vi "Write Registration Complete.vi"(8 "error in":errorcluster, 10 "Registration Complete":bool, 11 "File Actor in":refnum<class "File Actor.lvclass">) -> (0 "error out":errorcluster, 3 "File Actor out":refnum<class "File Actor.lvclass">)   [LabVIEW 2017, in "File Library.lvlib" / "File Actor.lvclass"]
doc: "Registers whether all data emitters have shown up to the party. Once they are completely registered, the system will send a message to start a new file. If the system is configured to save on start up, then a new file will be opened and the the header will be written to that file."
uses:
  File Actor.lvclass
  C:/Program Files (x86)/National Instruments/LabVIEW 2017/vi.lib/ActorFramework/Actor/Actor.lvclass
  File Actor.lvclass/File Actor.ctl
  Messages/To/Change File MSG/Change File MSG.lvclass
  C:/Program Files (x86)/National Instruments/LabVIEW 2017/vi.lib/ActorFramework/Message/Message.lvclass
  <vilib>/ActorFramework/Actor/Actor.lvclass/Actor.ctl
  <vilib>/ActorFramework/Message Enqueuer/Message Enqueuer.lvclass/Message Enqueuer.ctl
  <vilib>/ActorFramework/Message Enqueuer/Init from Existing Queue.vi
  <vilib>/ActorFramework/Message Priority Queue/Priority Enqueue.vi
  <vilib>/ActorFramework/Message Enqueuer/Message Enqueuer.lvclass
  <vilib>/ActorFramework/Actor/Actor.lvclass
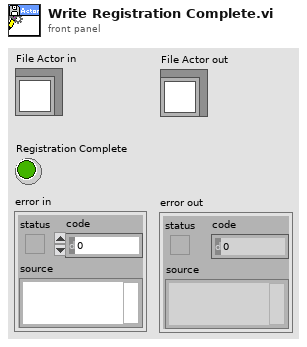
[diagram p1: front panel]
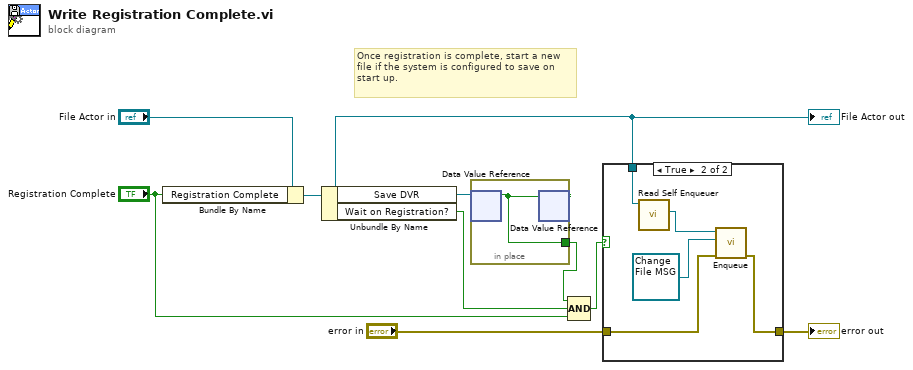
[diagram p0: block diagram]
diagram:
  # "Once registration is complete, start a new file if the system is configured to save on start up."
  n1 = Bundle By Name(cluster="File Actor in", "Registration Complete"="Registration Complete") -> (w7:refnum<class "File Actor.lvclass">)
  "File Actor out" <- w7
  n2 = Unbundle By Name(w7) -> ("Save DVR"=w8:refnum<data-value>, "Wait on Registration?"=w3:bool)
  n3 = in-place {
    in-place-border: [w10] -> w4
    n4 = in-place-dvr #1(w8) -> (w10:bool)  [unwired: 1 out]
    n5 = in-place-dvr #1(w10) -> ()  [unwired: 2 out]
  }
  n6 = Compound Arithmetic op=AND(w4, w3, "Registration Complete") -> (w1:bool)
  n7 = case shown="True" w1 {
    tunnel: w7 -> [_ w16]
    tunnel: "error in" -> [w11 w13]
    tunnel: [w11 w12] -> w5
    frame False {
    }
    frame True {
      n8 = call <vilib>:"Read Self Enqueuer.vi"("Actor"=w16) -> ("Self Enqueuer"=w14:refnum<class "Message Enqueuer.lvclass">)  [unwired: 10 in]
      n9 = call <vilib>:"Enqueue.vi"("error in (no error)"=w13, "Message"=refnum<class "Change File MSG.lvclass"> refnum ("File Library.lvlib:Change File MSG"), "Message Enqueuer in"=w14) -> ("error out"=w12:errorcluster)  [unwired: 7 in, 1 out]
    }
  }
  "error out" <- w5
